vi "Data To SingleElementsArray_with_itself_csm.vi"(6 "Seperator(/)":string="/", 8 "error in (no error)":errorcluster, 10 "parentUrl":string, 11 "Cluster":variant) -> (0 "error out":errorcluster, 2 "Full NameList":string[](array[string]), 3 "DataElementArray":variant[](array[variant]))   [LabVIEW 2017, in "API String Arguments Support.lvlib"]
doc: "This VI converts a Cluster to a DataElementArray with each elements specified by parentUrl and Seperator in the form of Tree Description."
uses:
  API String Arguments Support.lvlib
  <vilib>/Utility/Data Type/NI_Data Type.lvlib
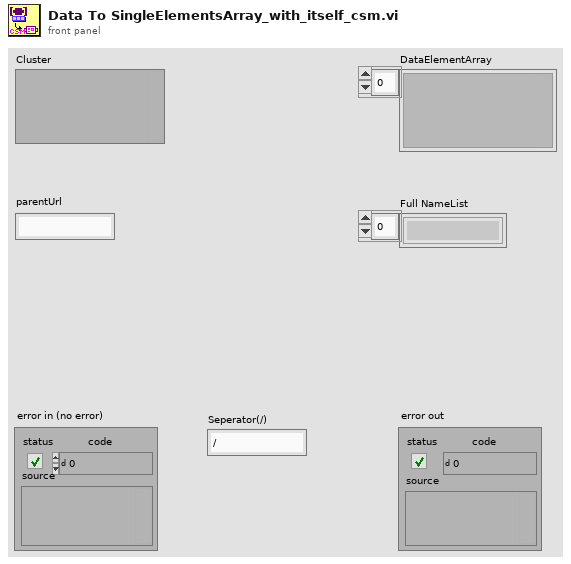
[diagram p1: front panel]
types:
  T1 = typedef "NI_Data Type.lvlib/Data Type.ctl" = enum8{"Invalid Type", "Void", "I8", "I16", "I32", "I64", "U8", "U16", "U32", "U64", "Single Float", "Double Float", "Extended Float", "Single Complex", "Double Complex", "Extended Complex", "Enum U8", "Enum U16", "Enum U32", "Enum U64", "Single Float With Unit", "Double Float With Unit", "Extended Float With Unit", "Single Complex with Unit", "Double Complex with Unit", "Extended Complex with Unit", "Boolean", "String", "Path", "Picture", "Tag", "Array", "Cluster", "Variant", "LV Variant", "Waveform", "Timestamp", "Digital Waveform", "Digital Data", "ExpressData", "Refnum", "External Data", "VI", "Poly VI", "LabVIEW Class Instance", "Fixed Point"}
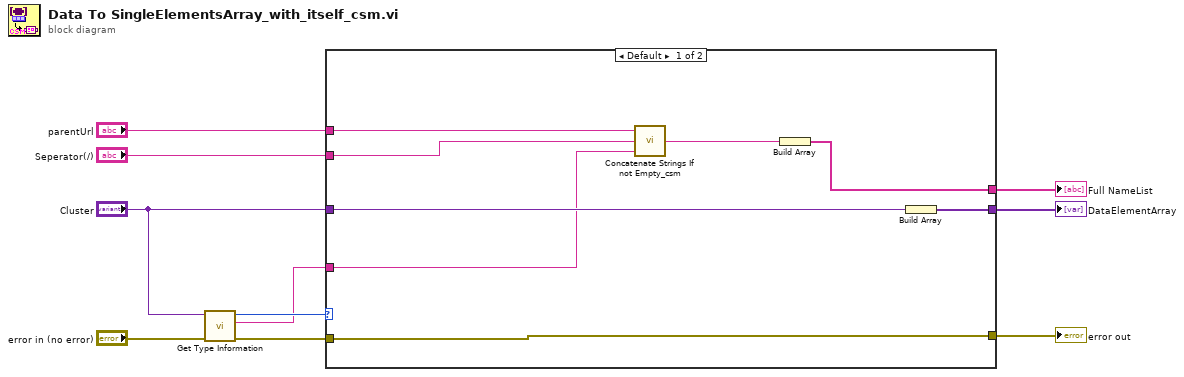
[diagram p0: block diagram]
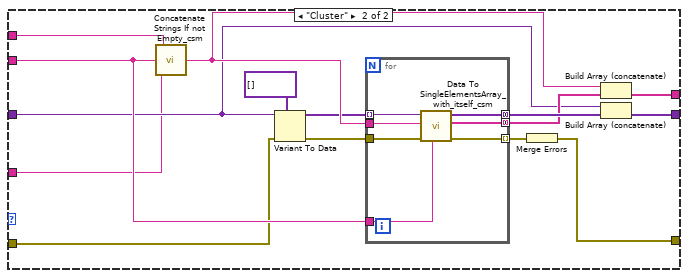
[diagram p2: hidden frame]
diagram:
  n1 = call <vilib>:"Get Type Information.vi"("error in (no error)"="error in (no error)", "Variant"="Cluster") -> ("error out"=w4:errorcluster, "Name"=w1:string, "Type"=w2:T1)  [unwired: 5 in, 2 out]
  n2 = case shown="Default" w2 {
    tunnel: "Cluster" -> [w12 w20]
    tunnel: "parentUrl" -> [w18 w31]
    tunnel: w4 -> [w13 w21]
    tunnel: [w13 w32] -> w8
    tunnel: [w17 w26] -> w7
    tunnel: [w15 w28] -> w6
    tunnel: "Seperator(/)" -> [w14 w27]
    tunnel: w1 -> [w11 w19]
    frame Default {
      n3 = call "Concatenate Strings If not Empty_csm.vi"("String"=w11, "seperator(:)"=w14, "prefix"=w18) -> ("result"=w16:string)  [unwired: 2 in]
      n4 = Build Array(w16) -> (w15:string[])
      n5 = Build Array(w12) -> (w17:variant[])
    }
    frame "Cluster" {
      n6 = call "Concatenate Strings If not Empty_csm.vi"("String"=w19, "seperator(:)"=w27, "prefix"=w31) -> ("result"=w25:string)  [unwired: 2 in]
      n7 = Variant To Data(error in=w21, type=variant[] [] ("Array"), Variant=w20) -> (data=w23:variant[], error out=w22:errorcluster)
      n8 = for {
        tunnel: w23 -> [w40] mode=indexing
        tunnel: w25 -> [w39]
        tunnel: [w38] -> w30 mode=concatenating
        tunnel: w22 -> [w37]
        tunnel: [w36] -> w33 mode=indexing
        tunnel: [w35] -> w29 mode=concatenating
        tunnel: w27 -> [w34]
        n9 = call "Data To SingleElementsArray_with_itself_csm.vi"("Seperator(/)"=w34, "error in (no error)"=w37, "parentUrl"=w39, "Cluster"=w40) -> ("error out"=w36:errorcluster, "Full NameList"=w35:string[], "DataElementArray"=w38:variant[])  [unwired: 5 in]
      }
      n10 = Merge Errors(w33) -> (w32:errorcluster)
      n11 = Build Array (concatenate)(w25, w29) -> (w28:string[])
      n12 = Build Array (concatenate)(w20, w30) -> (w26:variant[])
    }
  }
  "Full NameList" <- w6
  "error out" <- w8
  "DataElementArray" <- w7
